vi "Module Type.vi"(11 "DAQmxAI in":refnum<class "DAQmxAI.lvclass">) -> (2 "Module Type":string)   [LabVIEW 2020, in "VolatusDAQ.lvlib" / "DAQmxAI.lvclass"]
uses:
  DAQmxAI.lvclass
  DAQmxAI.lvclass/DAQmxAI.ctl
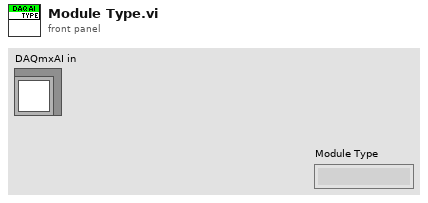
[diagram p1: front panel]
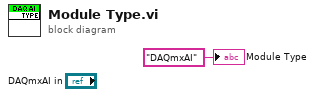
[diagram p0: block diagram]
diagram:
  "Module Type" <- "DAQmxAI" ("Module Type")
